vi "chart series set trendline line.vi"(8 "error in (no error)":errorcluster, 10 "line":T1, 11 "series":u32) -> (0 "error out":errorcluster, 2 "line out":T1)   [LabVIEW 8.6]
doc: "void chart_series_set_trendline_line(lxw_chart_series series, lxw_chart_line *line);"
uses:
  pending_lvxlsxwriter/xlsxwriter.dll
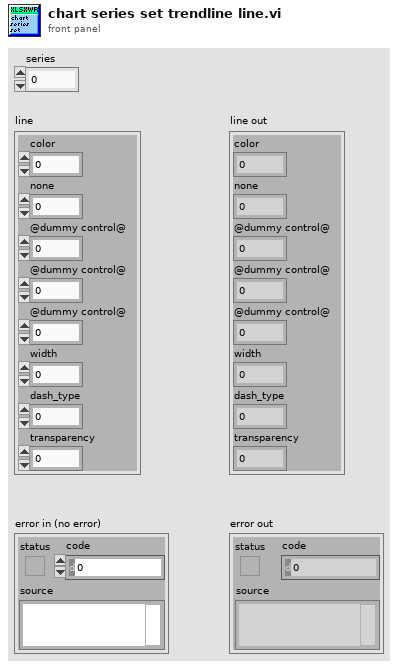
[diagram p1: front panel]
types:
  T1 = cluster{"color":u32, "none":u8, "@dummy control@":i8, "@dummy control@":i8, "@dummy control@":i8, "width":sgl, "dash_type":u8, "transparency":u8}
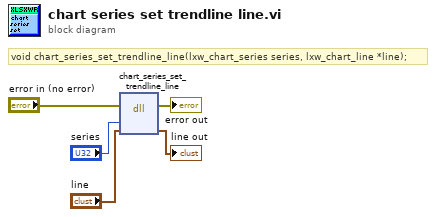
[diagram p0: block diagram]
diagram:
  # "void chart_series_set_trendline_line(lxw_chart_series series, lxw_chart_line *line);"
  n1 = dll-call lib="C:/Users/WDAGUtilityAccount/Desktop/pending_lvxlsxwriter/xlsxwriter.*" fn="chart_series_set_trendline_line"(error in="error in (no error)", "series"="series", "line"="line") -> (error out=→"error out":errorcluster, "line"=→"line out":T1)  [unwired: 4 in, 1 out]
